vi "Release.vi"   [LabVIEW 2021]
uses:
  AES/AES.lvclass
  RSA/RSA.lvclass
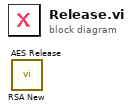
[diagram p0: block diagram]
diagram:
  n1 = call "RSA New.vi"() -> ()  [unwired: 10 in, 2 out]
  n2 = call "AES Release.vi"() -> ()  [unwired: 11 in, 1 out]
